vi "Set Chain Message.vi"(6 "Separator (-)":string=" - ", 7 "Msg Chain":string, 8 "error in (no error)":errorcluster {"code" format="Error %.0f"}, 10 "New":string, 11 "VIDoc Printer In":refnum<class "VIDoc Printer.lvclass">) -> (0 "error out":errorcluster {"code" format="Error %.0f"}, 3 "VIDoc Printer Out":refnum<class "VIDoc Printer.lvclass">, 5 "Msg Chain out":string)   [LabVIEW 2023, in "VIDoc Printer.lvlib" / "VIDoc Printer.lvclass"]
uses:
  VIDoc Printer.lvclass
  VIDoc Printer.lvclass/VIDoc Printer.ctl
  UI Interaction/UI Interaction.lvclass
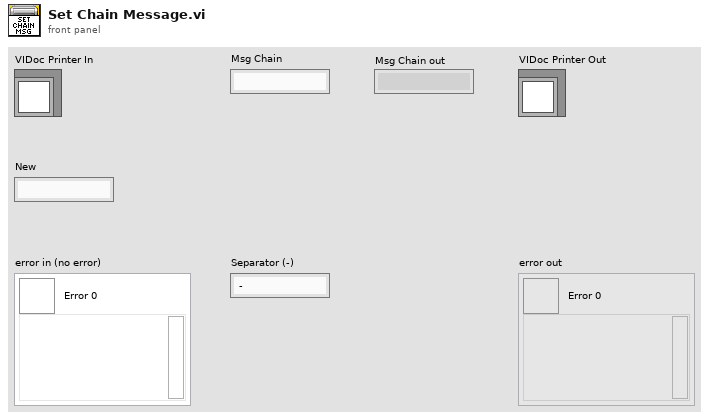
[diagram p1: front panel]
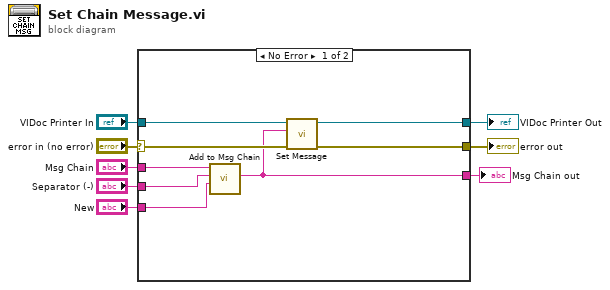
[diagram p0: block diagram]
diagram:
  n1 = case shown="No Error" "error in (no error)" {
    selector: "error in (no error)" -> [w11 w18]
    tunnel: [w10 w18] -> w7
    tunnel: [w12 w17] -> w5
    tunnel: "VIDoc Printer In" -> [w13 w17]
    tunnel: "New" -> [w16 _]
    tunnel: "Msg Chain" -> [w15 _]
    tunnel: "Separator (-)" -> [w14 _]
    tunnel: [w9 _] -> w1
    frame No Error {
      n2 = call "Add to Msg Chain.vi"("New"=w16, "Separator (-)"=w14, "Msg Chain in"=w15) -> ("Msg Chain out"=w9:string)  [unwired: 8 in]
      n3 = call "Set Message.vi"("error in (no error)"=w11, "Message"=w9, "VIDoc Printer In"=w13) -> ("error out"=w10:errorcluster, "VIDoc Printer Out"=w12:refnum<class "VIDoc Printer.lvclass">)  [unwired: 7 in]
    }
    frame Error {
    }
  }
  "error out" <- w7
  "VIDoc Printer Out" <- w5
  "Msg Chain out" <- w1
